vi "KepcoDCPwr Arbitrary Waveform.vi"(0 "VISA resource name":refnum<visa-resource-name>="GPIB0::3::INSTR", 1 "Open / Close":bool=TRUE, 5 "Model In":string, 11 "error in (no error)":errorcluster) -> (15 "error out":errorcluster)   [LabVIEW 2013]
panel:
  out "List not\nCorrected":bool
  out "list run":bool=TRUE
  out "Download time":u32
  out "Total time 2":dbl
  in  "CLR LIST":bool
  out "Total time":dbl=0.0015
  out "Measured Voltage Outptut":dbl(graph)=0.0646 caption="Current Measurements"
  in  "Load CSV":bool
  in  "List type":bool=TRUE
  out "Instrument Error":errorcluster
  in  "Start":bool caption="Downloading"
  in  "Exit":bool
  in  "Stop":bool
  in  "Protect":dbl caption="Voltage" min=0.0 max=20.0 step=1.0 format="%.2f"
  in  "Waveform List":string[][](table)=[["1", ".01"], ["2", ".01"], ["3", ".01"], ["4\n", ".01"], ["3", ".01"], ["2", ".01"], ["1", ".01"], ["0", ".01"]]
  in  "# of Cycles":i32=1
  in  "Disable @ End":bool
  out "Waveform Graph":T1(graph)={"Dwell (Sec)"=[0.0, 0.0005, 0.001, 0.0015], "Voltage Data"=[1.0, 2.0, 3.0]}
  out "number of points":i32=3 caption="Number of points"
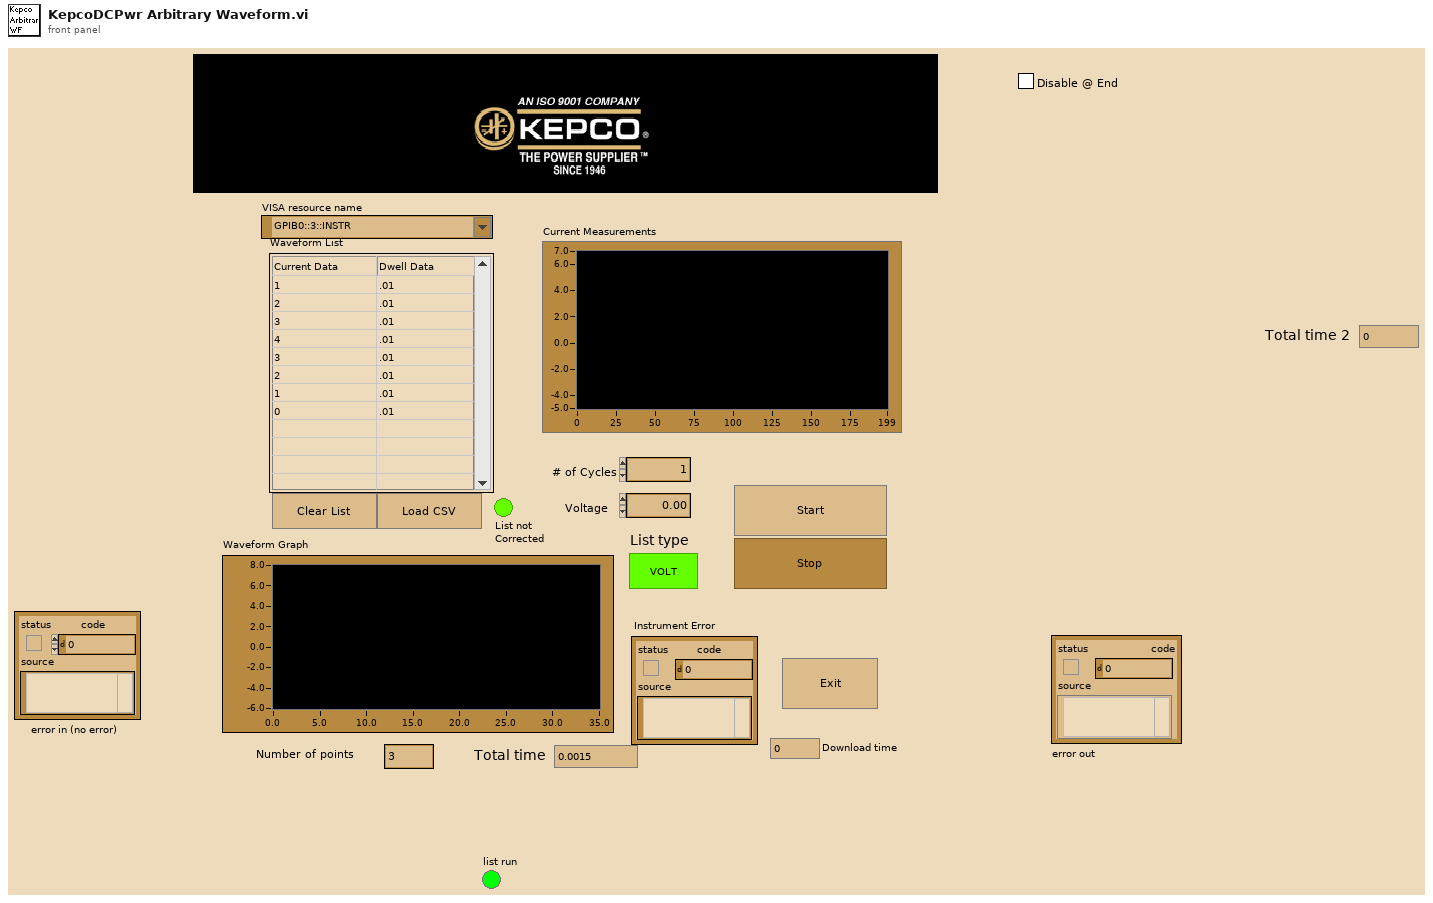
[diagram p1: front panel]
types:
  T1 = cluster{"Dwell (Sec)":dbl[], "Voltage Data":dbl[]}
  T2 = cluster{bool, "error code":i32, "error message":string}
  T3 = enum16{"Fixed", "List", "Transient", "External", "Gain", "Protect"}
  T4 = enum16{"open", "replace", "create", "open or create", "replace or create", "replace or create with confirmation"}
  T5 = cluster{"[0]":i32, "[1]":i32, "[2]":i32, "[3]":i32, "[4]":i32, "[5]":i32, "[6]":i32, "[7]":i32, "[8]":i32}
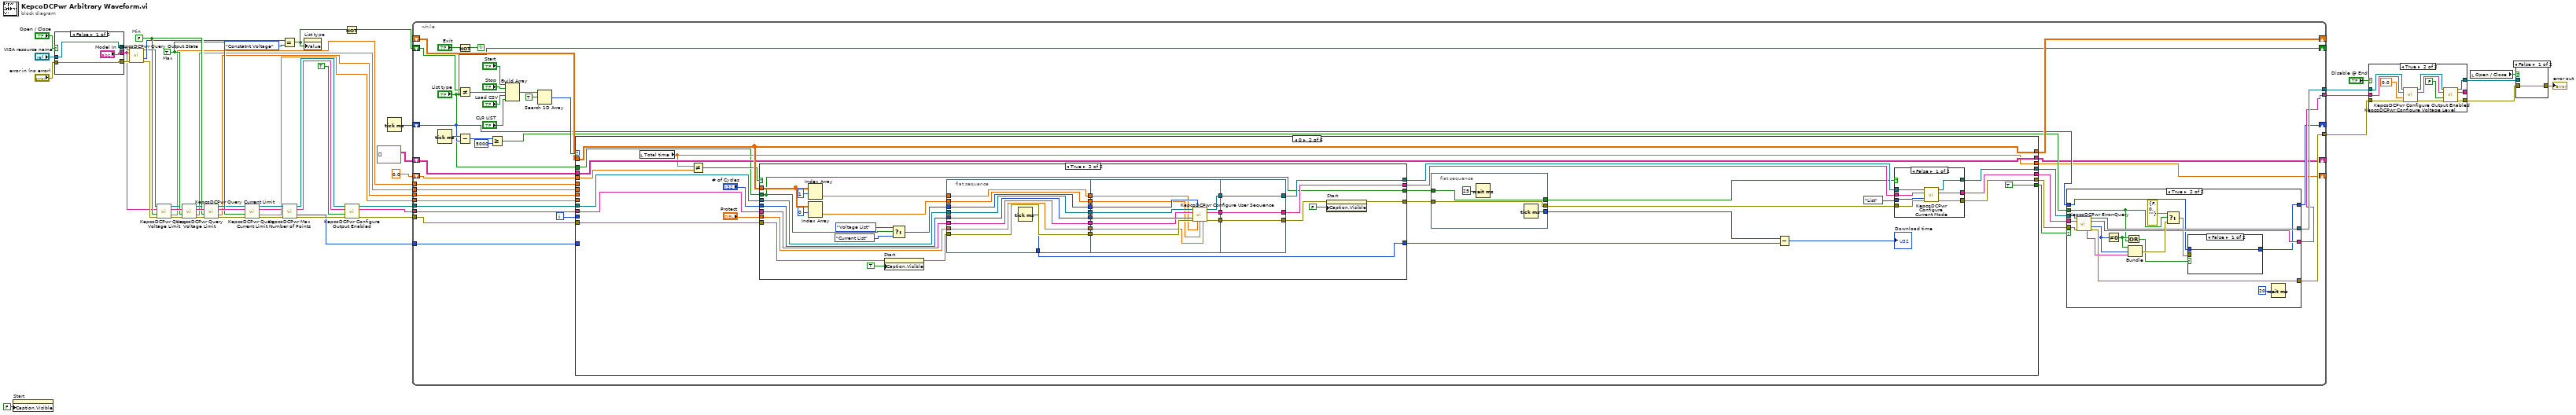
[diagram p0: block diagram]
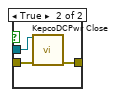
[diagram p2: hidden frame]
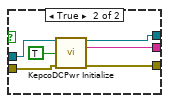
[diagram p3: hidden frame]
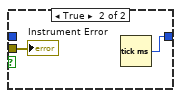
[diagram p5: hidden frame]
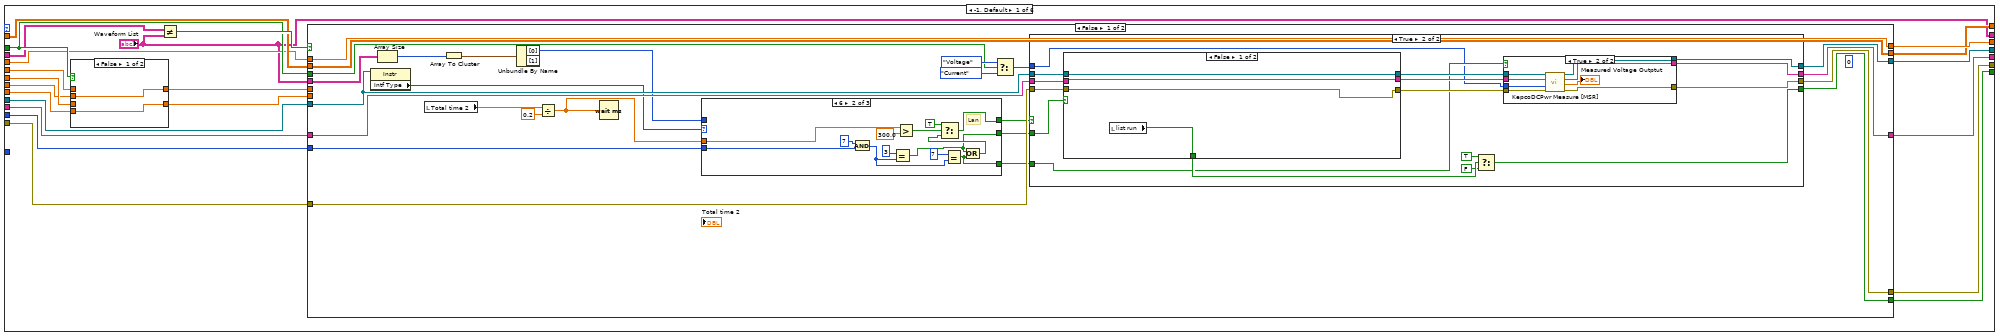
[diagram p6: hidden frame]
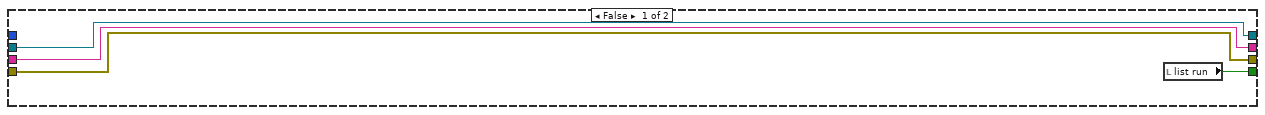
[diagram p8: hidden frame]
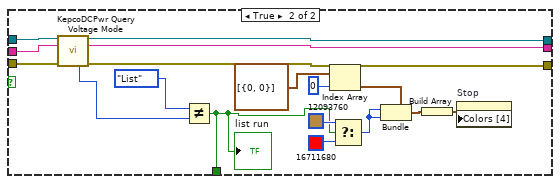
[diagram p9: hidden frame]
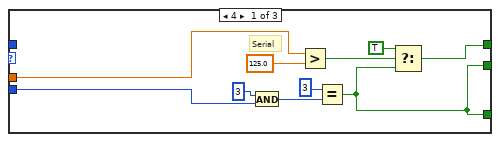
[diagram p11: hidden frame]
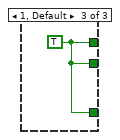
[diagram p12: hidden frame]
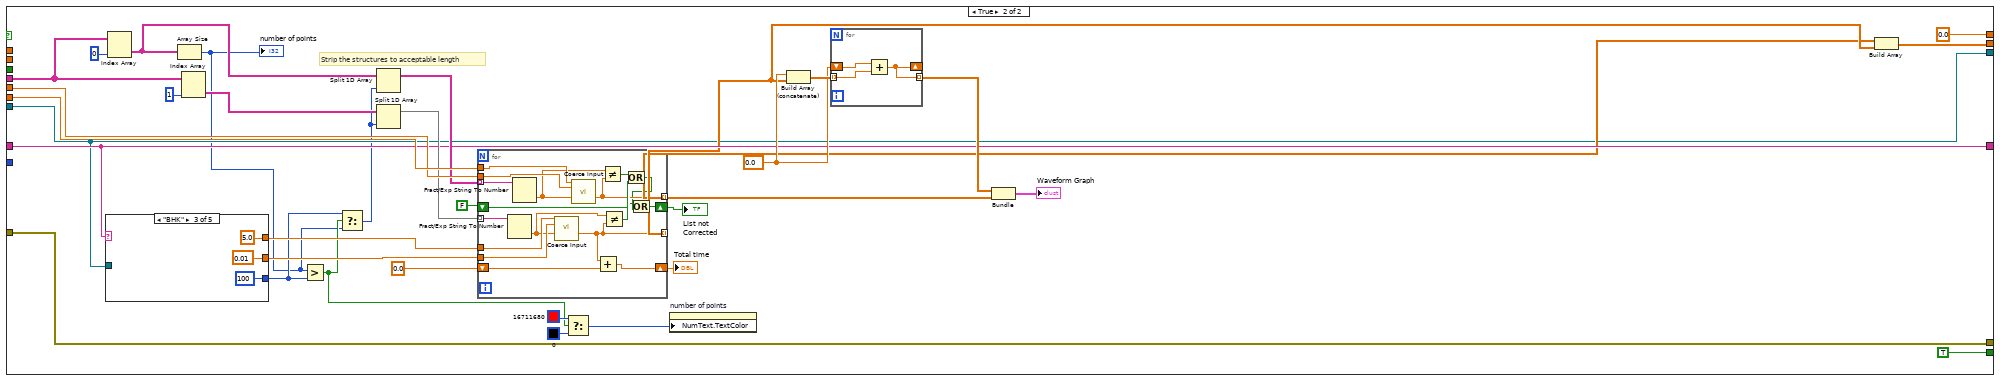
[diagram p13: hidden frame]
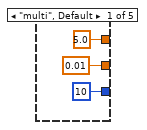
[diagram p14: hidden frame]
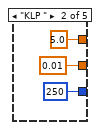
[diagram p15: hidden frame]
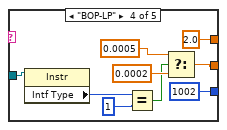
[diagram p16: hidden frame]
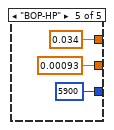
[diagram p17: hidden frame]
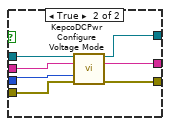
[diagram p18: hidden frame]
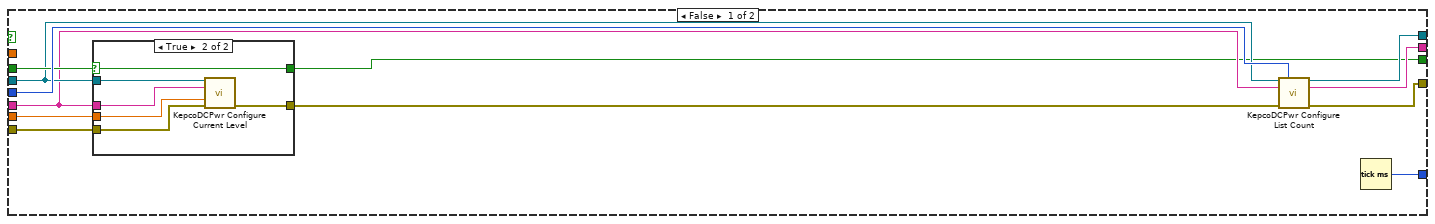
[diagram p19: hidden frame]
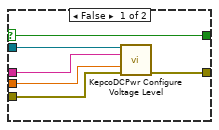
[diagram p20: hidden frame]
diagram:
  w26 = TRUE  # Max
  w27 = FALSE  # Min
  n1 = property on="Start" class="Bool"("Caption.Visible"=FALSE) -> ()  [unwired: 2 in, 2 out]
  n2 = case shown="False" "Open / Close" {
    tunnel: "error in (no error)" -> [w52 w58]
    tunnel: "VISA resource name" -> [w53 w57]
    tunnel: [w52 w56] -> w14
    tunnel: [w53 w55] -> w12
    tunnel: ["Model In" w54] -> w10
    frame False {
    }
    frame True {
      n3 = call "KepcoDCPwr Initialize.vi"("VISA Resource Name"=w57, "id query (True)"=TRUE, "error in (no error)"=w58) -> ("VISA Session Out"=w55:refnum<visa-resource-name>, "Model Out"=w54:string, "error out"=w56:errorcluster)  [unwired: 3 in, 7 out]
    }
  }
  n4 = call "KepcoDCPwr Query Output State.vi"("VISA Session"=w12, "Model In"=w10, "error in (no error)"=w14) -> ("VISA Session Out"=w11:refnum<visa-resource-name>, "Output state (Constant Voltage)"=w15:enum16{"Constatnt Voltage", "Constant Current"}, "error out"=w13:errorcluster)  [unwired: 5 in, 5 out]
  n5 = call "KepcoDCPwr Query Voltage Limit.vi"("VISA Session"=w11, "Model In"=w10, "Max Level (T),MIN LEVEL(F)"=w27, "error in (no error)"=w13) -> ("VISA Session Out"=w23:refnum<visa-resource-name>, "Model Out"=w32:string, "voltage level"=w17:dbl, "error out"=w33:errorcluster)  [unwired: 1 in, 7 out]
  n6 = call "KepcoDCPwr Query Voltage Limit.vi"("VISA Session"=w23, "Model In"=w32, "Max Level (T),MIN LEVEL(F)"=w26, "error in (no error)"=w33) -> ("VISA Session Out"=w24:refnum<visa-resource-name>, "Model Out"=w28:string, "voltage level"=w18:dbl, "error out"=w31:errorcluster)  [unwired: 1 in, 7 out]
  n7 = call "KepcoDCPwr Query Current Limit.vi"("VISA Session"=w24, "Model In"=w28, "Level"=w27, "error in (no error)"=w31) -> ("VISA Session Out"=w25:refnum<visa-resource-name>, "Model Out"=w29:string, "current limit"=w19:dbl, "error out"=w30:errorcluster)  [unwired: 1 in, 7 out]
  n8 = call "KepcoDCPwr Query Current Limit.vi"("VISA Session"=w25, "Model In"=w29, "Level"=w26, "error in (no error)"=w30) -> ("VISA Session Out"=w21:refnum<visa-resource-name>, "Model Out"=w7:string, "current limit"=w20:dbl, "error out"=w22:errorcluster)  [unwired: 1 in, 7 out]
  n9 = Equal?(x=w15, y=enum16{"Constatnt Voltage", "Constant Current"}."Constatnt Voltage" ("Output state (Constant Voltage)")) -> (x = y?=w9:bool)
  n10 = call "KepcoDCPwr Max Number of Points.vi"("VISA Session"=w21, "Model In"=w7, "error in (no error)"=w22) -> ("VISA Session Out"=w36:refnum<visa-resource-name>, "Model Out"=w34:string, "Max # of Pts"=w1:i32, "error out"=w35:errorcluster)  [unwired: 1 in, 8 out]
  n11 = property on="List type" class="Bool (strict)"("Value"=w9) -> ()  [unwired: 2 in, 2 out]
  n12 = Not(x=w9) -> (.not. x?=w8:bool)
  n13 = call "KepcoDCPwr Configure Output Enabled.vi"("VISA Session"=w36, "Model In"=w34, "Input enabled (True)"=TRUE, "error in (no error)"=w35) -> ("VISA Session Out"=w46:refnum<visa-resource-name>, "Model Out"=w45:string, "error out"=w44:errorcluster)  [unwired: 9 out]
  n14 = Tick Count (ms)() -> (millisecond timer value=w38:u32)
  n15 = while {
    shift-left: w38 -> [w78]
    shift-right: [w76] -> _
    shift-left: _ -> [w92]
    shift-right: [w91] -> _
    tunnel: w44 -> [w98]
    tunnel: [w82] -> w41
    tunnel: w45 -> [w97]
    tunnel: [w81] -> w42
    tunnel: w46 -> [w96]
    tunnel: [w83] -> w43
    shift-right: ["List type"] -> _
    shift-left: w8 -> [w75]
    tunnel: w19 -> [w71]
    tunnel: w20 -> [w70]
    tunnel: w18 -> [w72]
    tunnel: w17 -> [w73]
    shift-right: [w69] -> _
    shift-left: string[][] [] ("Data Table") -> [w68]
    shift-right: [w65] -> _
    shift-left: 0.0 ("Total time") -> [w64]
    tunnel: w1 -> [w60]
    i -> [w62]
    stop <- w99 continue-if-true
    n16 = Tick Count (ms)() -> (millisecond timer value=w87:u32)
    n17 = Not(x="Exit") -> (.not. x?=w99:bool)
    n18 = Not Equal?(x=w75, y="List type") -> (x != y?=w74:bool)
    n19 = Subtract(x=w87, y=w78) -> (x-y=w86:u32)
    n20 = Greater Or Equal?(x=w86, y=u32 5000) -> (x >= y?=w77:bool)
    n21 = Build Array("Start", "Stop", w74, "Load CSV", "CLR LIST") -> (w95:bool[])
    n22 = Search 1D Array(1D array=w95, element=TRUE) -> (index of element=w94:i32)  [unwired: 1 in]
    n23 = case shown="0" w94 {
      tunnel: w96 -> [w142 w342 w468 w501 w519 w542]
      tunnel: w97 -> [w141 w343 w467 w499 w520 w540]
      tunnel: w98 -> [w140 w344 w451 w498 w521 w538]
      tunnel: [w138 w349 w468 w500 w519 w541] -> w84
      tunnel: w92 -> [w144 w345 w469 w495 w524 w546]
      tunnel: [w136 w345 w469 w495 w524 w546] -> w91
      tunnel: [w139 w333 w450 w496 w521 w537] -> w80
      tunnel: [w137 w350 w467 w497 w520 w539] -> w79
      tunnel: w73 -> [w134 _ _ _ _ w536]
      tunnel: w72 -> [w133 _ _ _ _ w535]
      tunnel: w71 -> [w132 _ _ _ _ w533]
      tunnel: w70 -> [w131 _ _ _ _ w532]
      tunnel: ["Waveform List" w341 w453 w494 w523 string[][] [] ("Data Table")] -> w69
      tunnel: w68 -> [w126 w341 w453 w494 w523 _]
      tunnel: "List type" -> [w135 w336 _ w492 _ w529]
      tunnel: [w143 w340 w452 w493 w522 w531] -> w65
      tunnel: w64 -> [w128 w339 w452 w493 w522 w531]
      tunnel: w62 -> [w125 _ _ _ _ _]
      tunnel: [w124 TRUE _ TRUE TRUE TRUE] -> w61
      tunnel: w60 -> [_ _ _ _ _ _]
      frame -1, Default {
        n24 = case shown="False" w135 {
          tunnel: w134 -> [_ w149]
          tunnel: w133 -> [_ w148]
          tunnel: w132 -> [w147 _]
          tunnel: w131 -> [w146 _]
          tunnel: [w147 w149] -> w129
          tunnel: [w146 w148] -> w130
          frame False {
          }
          frame True {
          }
        }
        n25 = Not Equal?(x=w126, y="Waveform List") -> (x != y?=w145:bool)
        n26 = case shown="False" w145 {
          tunnel: [w174 w259] -> w136
          tunnel: w130 -> [_ w284]
          tunnel: w129 -> [_ w283]
          tunnel: "Waveform List" -> [w160 w267]
          tunnel: w144 -> [w174 _]
          tunnel: [w163 0.0 ("Total time")] -> w143
          tunnel: w135 -> [w171 _]
          tunnel: w142 -> [w162 w255]
          tunnel: w141 -> [w170 w264]
          tunnel: w140 -> [w169 w265]
          tunnel: [w167 w265] -> w139
          tunnel: [w166 w255] -> w138
          tunnel: [w165 w264] -> w137
          tunnel: w128 -> [w163 _]
          tunnel: w125 -> [w155 _]
          tunnel: [w152 TRUE] -> w124
          frame False {
            (unwired) 0 ("y")
            n27 = property class="Instr"(reference=w162) -> ("Intf Type"=w161:u16)  [unwired: 1 in, 2 out]
            n28 = Array Size(array=w160) -> (size(s)=w159:i32[])
            n29 = local read "Total time 2"() -> (w164:dbl)
            n30 = Array To Cluster(array=w159) -> (cluster=w158:T5)
            n31 = Unbundle By Name(w158) -> ("[0]"=w157:i32)  [unwired: 1 out]
            n32 = Divide(x=w164, y=0.2) -> (x/y=w153:dbl)
            n33 = Wait (ms)(milliseconds to wait=w153) -> ()  [unwired: 1 out]
            n34 = case shown="6" w161 {
              tunnel: w157 -> [_ _ _]
              tunnel: [w229 w243 w250] -> w156
              tunnel: w155 -> [w236 w249 _]
              tunnel: w153 -> [w232 w246 _]
              tunnel: [w227 w238 w250] -> w151
              tunnel: [w227 w237 w250] -> w150
              frame 4 {
                # "Serial"
                n35 = And(x=3, y=w236) -> (x .and. y?=w234:i32)
                n36 = Greater?(x=w232, y=125.0) -> (0:w230:bool)
                n37 = Equal?(x=3, y=w234) -> (x = y?=w227:bool)
                n38 = Select(t=TRUE, s=w230, f=w227) -> (s? t:f=w229:bool)
              }
              frame 6 {
                # "Lan"
                n39 = And(x=7, y=w249) -> (x .and. y?=w241:i32)
                n40 = Equal?(x=3, y=w241) -> (x = y?=w238:bool)
                n41 = Greater?(x=w246, y=300.0) -> (0:w244:bool)
                n42 = Equal?(x=7, y=w241) -> (x = y?=w237:bool)
                n43 = Or(x=w238, y=w237) -> (x .or. y?=w239:bool)
                n44 = Select(t=TRUE, s=w244, f=w239) -> (s? t:f=w243:bool)
              }
              frame 1, Default {
                w250 = TRUE
              }
            }
            n45 = Select(t=enum16{"Voltage", "Current"}."Voltage" ("measurement type (voltage)"), s=w171, f=enum16{"Voltage", "Current"}."Current") -> (s? t:f=w168:enum16{"Voltage", "Current"})
            n46 = case shown="True" w156 {
              tunnel: w170 -> [w177 w191]
              tunnel: w169 -> [w176 w190]
              tunnel: w168 -> [_ w179]
              tunnel: [w176 w189] -> w167
              tunnel: [w178 w188] -> w166
              tunnel: [w177 w187] -> w165
              tunnel: w162 -> [w178 w186]
              tunnel: [w175 w183] -> w152
              tunnel: w151 -> [_ w181]
              tunnel: w150 -> [_ w180]
              frame False {
                n47 = local read "list run"() -> (w175:bool)
              }
              frame True {
                n48 = case shown="False" w181 {
                  tunnel: [w196 w207] -> w194
                  tunnel: [w195 w206] -> w193
                  tunnel: [w197 w205] -> w192
                  tunnel: w191 -> [w196 w204]
                  tunnel: w190 -> [w197 w203]
                  tunnel: w186 -> [w195 w202]
                  tunnel: [w198 w199] -> w185
                  frame False {
                    n49 = local read "list run"() -> (w198:bool)
                  }
                  frame True {
                    n50 = call "KepcoDCPwr Query Voltage Mode.vi"("VISA Session"=w202, "Model In"=w204, "error in (no error)"=w203) -> ("VISA Session Out"=w206:refnum<visa-resource-name>, "Model Out"=w207:string, "Mode (Fixed)"=w201:T3, "error out"=w205:errorcluster)  [unwired: 1 in, 8 out]
                    n51 = Not Equal?(x=T3."List", y=w201) -> (x != y?=w199:bool)
                    "list run" <- w199
                    n52 = Index Array(array=cluster{u32, u32}[] [{0, 0}] ("Colors [4]"), index=0) -> (element=w213:cluster{u32, u32})
                    n53 = Select(t=u32 12093760, s=w199, f=u32 16711680) -> (s? t:f=w210:u32)
                    n54 = Bundle(cluster=w213, w210, w210) -> (w212:cluster{u32, u32})
                    n55 = Build Array(w212) -> (w215:cluster{u32, u32}[])
                    n56 = property on="Stop" class="Bool"("Colors [4]"=w215) -> ()  [unwired: 2 in, 2 out]
                  }
                }
                n57 = Select(t=TRUE, s=w185, f=FALSE ("x != y?")) -> (s? t:f=w183:bool)
                n58 = case shown="True" w180 {
                  tunnel: w194 -> [w216 w226]
                  tunnel: w193 -> [w217 w225]
                  tunnel: w192 -> [w218 w224]
                  tunnel: w179 -> [_ w223]
                  tunnel: [w218 w221] -> w189
                  tunnel: [w217 w220] -> w188
                  tunnel: [w216 w219] -> w187
                  frame False {
                  }
                  frame True {
                    n59 = call "KepcoDCPwr Measure [MSR].vi"("VISA Session"=w225, "Model In"=w226, "measurement type (voltage)"=w223, "error in (no error)"=w224) -> ("VISA Session Out"=w220:refnum<visa-resource-name>, "Model Out"=w219:string, "measurement"=→"Measured Voltage Outptut":dbl, "error out"=w221:errorcluster)  [unwired: 4 in, 4 out]
                  }
                }
              }
            }
          }
          frame True {
            w279 = 0.0
            # "Strip the structures to acceptable length"
            n60 = case shown="\"BHK\"" w264 {
              tunnel: [5.0 5.0 5.0 2.0 0.034] -> w263
              tunnel: [0.01 0.01 0.01 w297 0.00093] -> w262
              tunnel: [10 250 100 1002 5900] -> w253
              tunnel: w255 -> [_ _ _ w300 _]
              frame "multi", Default {
              }
              frame "KLP " {
              }
              frame "BHK" {
              }
              frame "BOP-LP" {
                n61 = property class="Instr"(reference=w300) -> ("Intf Type"=w295:u16)  [unwired: 1 in, 2 out]
                n62 = Equal?(x=w295, y=u16 1 ("x")) -> (x = y?=w296:bool)
                n63 = Select(t=0.0005, s=w296, f=0.0002) -> (s? t:f=w297:dbl)
              }
              frame "BOP-HP" {
              }
            }
            n64 = Index Array(array=w267, index (col)=0) -> (element=w266:string[])  [unwired: 1 in]
            n65 = Array Size(array=w266) -> (size(s)=w252:i32)
            "number of points" <- w252
            n66 = Index Array(array=w267, index (col)=1) -> (element=w275:string[])  [unwired: 1 in]
            n67 = Greater?(x=w252, y=w253) -> (0:w254:bool)
            n68 = Select(t=w253, s=w254, f=w252) -> (s? t:f=w251:i32)
            n69 = Split 1D Array(array=w266, index=w251) -> (first subarray=w276:string[])  [unwired: 1 out]
            n70 = Split 1D Array(array=w275, index=w251) -> (first subarray=w274:string[])  [unwired: 1 out]
            n71 = for {
              tunnel: w276 -> [w322] mode=indexing
              tunnel: [w312] -> w260 mode=indexing
              tunnel: w274 -> [w321] mode=indexing
              tunnel: [w311] -> w261 mode=indexing
              tunnel: w284 -> [w313]
              tunnel: w283 -> [w320]
              shift-right: [w319] -> w272
              shift-left: 0.0 -> [w318]
              tunnel: w263 -> [w317]
              tunnel: w262 -> [w316]
              shift-right: [w306] -> w256
              shift-left: FALSE -> [w307]
              n72 = Fract/Exp String To Number(string=w321) -> (number=w309:dbl)  [unwired: 4 out]
              n73 = Fract/Exp String To Number(string=w322) -> (number=w310:dbl)  [unwired: 4 out]
              n74 = call "Coerce Input.vi"("Max"=w317, "Min"=w316, "Input"=w309) -> ("Output"=w311:dbl)  [unwired: 12 out]
              n75 = call "Coerce Input.vi"("Max"=w313, "Min"=w320, "Input"=w310) -> ("Output"=w312:dbl)  [unwired: 12 out]
              n76 = Add(x=w311, y=w318) -> (x+y=w319:dbl)
              n77 = Not Equal?(x=w310, y=w312) -> (x != y?=w315:bool)
              n78 = Not Equal?(x=w309, y=w311) -> (x != y?=w314:bool)
              n79 = Or(x=w315, y=w314) -> (x .or. y?=w308:bool)
              n80 = Or(x=w307, y=w308) -> (x .or. y?=w306:bool)
            }
            "Total time" <- w272
            "List not\nCorrected" <- w256
            n81 = Select(t=u32 16711680, s=w254, f=u32 0) -> (s? t:f=w270:u32)
            n82 = property on="number of points" class="DigNum (strict)"("NumText.TextColor"=w270) -> ()  [unwired: 2 in, 2 out]
            n83 = Build Array (concatenate)(w279, w261) -> (w280:dbl[])
            n84 = for {
              tunnel: w280 -> [w325] mode=indexing
              shift-right: [w323] -> _
              shift-left: w279 -> [w324]
              tunnel: [w323] -> w281 mode=indexing
              n85 = Add(x=w324, y=w325) -> (x+y=w323:dbl)
            }
            n86 = Bundle(w281, w260) -> (→"Waveform Graph":cluster{dbl[], dbl[]})  [unwired: 1 out]
            n87 = Build Array(w260, w261) -> (w259:dbl[][])
          }
        }
      }
      frame 0 {
        n88 = local read "Total time"() -> (w340:dbl)
        n89 = Not Equal?(x=w340, y=w339) -> (x != y?=w338:bool)
        n90 = case shown="True" w338 {
          tunnel: [w376 w421] -> w348
          tunnel: [w375 w420] -> w347
          tunnel: [w374 w413] -> w335
          tunnel: "# of Cycles" -> [w373 w419]
          tunnel: w345 -> [_ w405]
          tunnel: w344 -> [w368 w416]
          tunnel: w343 -> [w369 w418]
          tunnel: w342 -> [w370 w417]
          tunnel: "Protect" -> [w372 w410]
          tunnel: w336 -> [w371 w389]
          tunnel: [w366 w390] -> w330
          tunnel: [w365 w389] -> w328
          frame False {
            n91 = case shown="True" w371 {
              selector: w371 -> [w377 w383]
              tunnel: w372 -> [w382 w388]
              tunnel: w370 -> [w381 w387]
              tunnel: w369 -> [w380 w386]
              tunnel: w368 -> [w379 w384]
              tunnel: [w378 w385] -> w367
              tunnel: [w377 w383] -> w365
              frame False {
                n92 = call "KepcoDCPwr Configure Voltage Level.vi"("VISA Session"=w381, "Model In"=w380, "level (0.0 volts)"=w382, "error in (no error)"=w379) -> ("error out"=w378:errorcluster)  [unwired: 8 in, 3 out]
              }
              frame True {
                n93 = call "KepcoDCPwr Configure Current Level.vi"("VISA Session"=w387, "Model In"=w386, "level (0.0 volts)"=w388, "error in (no error)"=w384) -> ("error out"=w385:errorcluster)  [unwired: 8 in, 3 out]
              }
            }
            n94 = call "KepcoDCPwr Configure List Count.vi"("VISA Session"=w370, "# of Cycles"=w373, "Model In"=w369, "error in (no error)"=w367) -> ("VISA Session Out"=w376:refnum<visa-resource-name>, "Model Out"=w375:string, "error out"=w374:errorcluster)  [unwired: 8 in, 1 out]
            n95 = Tick Count (ms)() -> (millisecond timer value=w366:u32)
          }
          frame True {
            n96 = Index Array(array=w405, index (row)=1 ("index")) -> (element=w406:dbl[])  [unwired: 1 in]
            n97 = Index Array(array=w405, index (row)=0 ("index")) -> (element=w404:dbl[])  [unwired: 1 in]
            n98 = property on="Start" class="Bool"(error in=w416, "Caption.Visible"=TRUE) -> (error out=w415:errorcluster)  [unwired: 1 in, 1 out]
            n99 = Select(t=enum16{"Current List", "Voltage List"}."Voltage List" ("List Mode (volt/current)"), s=w389, f=enum16{"Current List", "Voltage List"}."Current List") -> (s? t:f=w408:enum16{"Current List", "Voltage List"})
            n100 = flat-sequence {
              tunnel: w404 -> [w423]
              tunnel: w406 -> [w424]
              tunnel: w408 -> [w425]
              tunnel: w410 -> [w426]
              tunnel: w415 -> [w427]
              tunnel: w417 -> [w428]
              tunnel: w418 -> [w429]
              tunnel: w419 -> [w430]
              tunnel: [w430] -> w398
              tunnel: [w429] -> w397
              tunnel: [w428] -> w396
              tunnel: [w427] -> w395
              tunnel: [w426] -> w394
              tunnel: [w425] -> w393
              tunnel: [w424] -> w392
              tunnel: [w423] -> w391
              tunnel: [w422] -> w390
              tunnel: [w441] -> w401
              tunnel: [w440] -> w400
              tunnel: [w435] -> w399
              tunnel: w398 -> [w439]
              tunnel: w397 -> [w438]
              tunnel: w396 -> [w437]
              tunnel: w395 -> [w436]
              tunnel: w394 -> [w434]
              tunnel: w393 -> [w433]
              tunnel: w392 -> [w432]
              tunnel: w391 -> [w431]
              tunnel: [w442] -> w412
              tunnel: [w443] -> w420
              tunnel: [w444] -> w421
              tunnel: w401 -> [w444]
              tunnel: w400 -> [w443]
              tunnel: w399 -> [w442]
              frame #0 {
                n101 = Tick Count (ms)() -> (millisecond timer value=w422:u32)
              }
              frame #1 {
                n102 = call "KepcoDCPwr Configure User Sequence.vi"("VISA Session"=w437, "List Mode (volt/current)"=w433, "Model In"=w438, "# of Cycles"=w439, "error in (no error)"=w436, "Dwell (sec)"=w432, "List Data"=w431, "Limit Value"=w434) -> ("VISA Session Out"=w441:refnum<visa-resource-name>, "Model Out"=w440:string, "error out"=w435:errorcluster)  [unwired: 1 in, 4 out]
              }
              frame #2 {
              }
            }
            n103 = property on="Start" class="Bool"(error in=w412, "Caption.Visible"=FALSE) -> (error out=w413:errorcluster)  [unwired: 1 in, 1 out]
          }
        }
        n104 = flat-sequence {
          tunnel: [w447] -> w334
          tunnel: w335 -> [w447]
          tunnel: [w446] -> w332
          tunnel: [w445] -> w329
          tunnel: w328 -> [w445]
          frame #0 {
            n105 = Wait (ms)(milliseconds to wait=u32 25) -> ()  [unwired: 1 out]
            n106 = Tick Count (ms)() -> (millisecond timer value=w446:u32)
          }
        }
        n107 = Subtract(x=w332, y=w330) -> (x-y=→"Download time":u32)
        n108 = case shown="False" w329 {
          tunnel: [w352 w364] -> w350
          tunnel: [w351 w363] -> w349
          tunnel: w348 -> [w357 w362]
          tunnel: w347 -> [w356 w361]
          tunnel: w334 -> [w355 w360]
          tunnel: [w353 w359] -> w333
          tunnel: T3."List" ("Mode (Fixed)") -> [w354 w358]
          frame False {
            n109 = call "KepcoDCPwr Configure Current Mode.vi"("VISA Session"=w357, "Model In"=w356, "Mode (Fixed)"=w354, "error in (no error)"=w355) -> ("VISA Session Out"=w351:refnum<visa-resource-name>, "Model Out"=w352:string, "error out"=w353:errorcluster)  [unwired: 8 in, 1 out]
          }
          frame True {
            n110 = call "KepcoDCPwr Configure Voltage Mode.vi"("VISA Session"=w362, "Model In"=w361, "Mode (Fixed)"=w358, "error in (no error)"=w360) -> ("VISA Session Out"=w363:refnum<visa-resource-name>, "Model Out"=w364:string, "error out"=w359:errorcluster)  [unwired: 2 in, 7 out]
          }
        }
      }
      frame 3 {
        n111 = Open/Create/Replace File(error in=w451, prompt="Select txt or csv file", operation (0:open)=T4."open", access (0:read/write)=enum16{"read/write", "read-only", "write-only"}."read-only") -> (refnum out=w461:refnum<file>, error out=w462:errorcluster)  [unwired: 2 in, 1 out]
        n112 = Get File Size(file=w461, error in=w462) -> (size (in bytes)=w456:i64, 0:w457:errorcluster)  [unwired: 1 out]
        n113 = while {
          tunnel: w461 -> [w477]
          tunnel: [w476] -> w460
          tunnel: [w471] -> w458
          tunnel: w457 -> [w470]
          stop <- w472 stop-if-true
          n114 = Read from Text File(file (use dialog)=w477, error in=w470) -> (refnum out=w476:refnum<file>, text=w475:string, error out=w471:errorcluster)  [unwired: 2 in, 1 out]
          n115 = Match Pattern(string=w475, regular expression="\"") -> (offset past match=w473:i32)  [unwired: 1 in, 3 out]
          n116 = Less Than 0?(x=w473) -> (x < 0?=w472:bool)
        }
        n117 = Subtract(x=w456, y=i64 5) -> (x-y=w454:i64)
        n118 = while {
          tunnel: w460 -> [w490]
          tunnel: [w485] -> w463
          tunnel: [w483] -> w459
          tunnel: w458 -> [w482]
          tunnel: w454 -> [w481]
          tunnel: [w478] -> w449 mode=indexing
          stop <- w487 stop-if-true
          n119 = Read from Text File(file (use dialog)=w490, error in=w482) -> (refnum out=w485:refnum<file>, text=w489:string, error out=w484:errorcluster)  [unwired: 2 in, 1 out]
          n120 = Get File Position(4:w484, 7:w485) -> (0:w483:errorcluster, 2:w486:i64)  [unwired: 1 out]
          n121 = Match Pattern(string=w489, regular expression="\t") -> (before substring=w480:string, after substring=w479:string)  [unwired: 1 in, 2 out]
          n122 = Greater?(x=w486, y=w481) -> (0:w487:bool)
          n123 = Build Array(w480, w479) -> (w478:string[])
        }
        n124 = local write "Waveform List"(w449) -> ()
        n125 = Close File(refnum=w463, error in=w459) -> (error out=w450:errorcluster)  [unwired: 1 out]
      }
      frame 1 {
        n126 = case shown="False" w492 {
          tunnel: T3."Fixed" ("Mode (Fixed)") -> [w509 w516]
          tunnel: w501 -> [w508 w515]
          tunnel: [w507 w514] -> w500
          tunnel: w499 -> [w506 w513]
          tunnel: w498 -> [w505 w512]
          tunnel: [w504 w511] -> w497
          tunnel: [w503 w510] -> w496
          frame False {
            n127 = call "KepcoDCPwr Configure Current Mode.vi"("VISA Session"=w508, "Model In"=w506, "Mode (Fixed)"=w509, "error in (no error)"=w505) -> ("VISA Session Out"=w507:refnum<visa-resource-name>, "Model Out"=w504:string, "error out"=w503:errorcluster)  [unwired: 8 in, 1 out]
          }
          frame True {
            n128 = call "KepcoDCPwr Configure Voltage Mode.vi"("VISA Session"=w515, "Model In"=w513, "Mode (Fixed)"=w516, "error in (no error)"=w512) -> ("VISA Session Out"=w514:refnum<visa-resource-name>, "Model Out"=w511:string, "error out"=w510:errorcluster)  [unwired: 2 in, 7 out]
          }
        }
      }
      frame 4 {
        # "Clear the waveform list"
        n129 = local write "Waveform List"(string[][] [["1", ".1"], ["2", ".1"]] ("Waveform List")) -> ()
      }
      frame 2 {
        # "List mode change"
        n130 = case shown="True" w529 {
          tunnel: w536 -> [_ _]
          tunnel: w535 -> [w550 _]
          tunnel: [w550 w554] -> w534
          tunnel: w533 -> [_ _]
          tunnel: w532 -> [_ w554]
          tunnel: ["Voltage" ("new element/subarray") "Current" ("f")] -> w528
          tunnel: ["Current Measurements" ("f") "Voltage Measurements" ("f")] -> w527
          tunnel: ["Current Data" ("f") "Voltage Data" ("new element/subarray")] -> w526
          frame False {
          }
          frame True {
          }
        }
        n131 = property on="Waveform List" class="Tbl (strict)"() -> ("Column Headers[]"=w545:string[])  [unwired: 2 in, 2 out]
        n132 = property on="Measured Voltage Outptut" class="WFChart (strict)"("Caption.Text"=w527) -> ()  [unwired: 2 in, 2 out]
        n133 = property on="Protect" class="DigNum (strict)"("Caption.Text"=w528, "Maximum"=w534) -> ()  [unwired: 2 in, 2 out]
        n134 = Replace Array Subset(array=w545, new element=w526, index=0) -> (w543:string[])
        n135 = property on="Waveform List" class="Tbl (strict)"("Column Headers[]"=w543) -> ()  [unwired: 2 in, 2 out]
        n136 = call "KepcoDCPwr Configure Output State.vi"("VISA Session"=w542, "Model In"=w540, "Power Supply Mode"=w529, "error in (no error)"=w538) -> ("VISA Session Out"=w541:refnum<visa-resource-name>, "channel name out (\"\")"=w539:string, "error out"=w537:errorcluster)  [unwired: 8 in, 1 out]
      }
    }
    n137 = case shown="True" w61 {
      tunnel: w84 -> [w103 w113]
      tunnel: [w103 w112] -> w83
      tunnel: [w100 w111] -> w82
      tunnel: [w101 w110] -> w81
      tunnel: w80 -> [w100 w109]
      tunnel: w79 -> [w101 w108]
      tunnel: w78 -> [w102 w107]
      tunnel: w77 -> [_ w106]
      tunnel: [w102 w105] -> w76
      frame False {
      }
      frame True {
        n138 = call "KepcoDCPwr Error-Query.vi"("VISA Session"=w113, "Model In"=w108, "error in (no error)"=w109) -> ("VISA Session Out"=w112:refnum<visa-resource-name>, "Model Out"=w110:string, "error code"=w116:i32, "error message"=w115:string, "error out"=w111:errorcluster)  [unwired: 1 in, 7 out]
        n139 = Not Equal To 0?(x=w116) -> (x != 0?=w117:bool)
        n140 = Or(x=w117, y=w106) -> (x .or. y?=w114:bool)
        n141 = Bundle(w117, "error code"=w116, "error message"=w115) -> (w118:T2)  [unwired: 1 out]
        n142 = Select(t=T2 {FALSE, "error code"=0, "error message"=""}, s=w106, f=w118) -> (s? t:f=w119:T2)
        n143 = case shown="False" w114 {
          tunnel: [w121 w123] -> w105
          tunnel: w107 -> [w121 _]
          tunnel: w119 -> [_ w122]
          frame False {
          }
          frame True {
            n144 = Tick Count (ms)() -> (millisecond timer value=w123:u32)
            "Instrument Error" <- w122
          }
        }
        n145 = Wait (ms)(milliseconds to wait=u32 20) -> ()  [unwired: 1 out]
      }
    }
  }
  n146 = case shown="True" "Disable @ End" {
    tunnel: w43 -> [w557 w568]
    tunnel: w42 -> [w556 w567]
    tunnel: w41 -> [w555 w566]
    tunnel: [w555 w561] -> w49
    tunnel: [w557 w560] -> w50
    tunnel: [w556 w559] -> _
    frame False {
    }
    frame True {
      n147 = call "KepcoDCPwr Configure Voltage Level.vi"("VISA Session"=w568, "Model In"=w567, "level (0.0 volts)"=0.0, "error in (no error)"=w566) -> ("VISA Session Out"=w564:refnum<visa-resource-name>, "Model Out"=w563:string, "error out"=w562:errorcluster)  [unwired: 1 in, 8 out]
      n148 = call "KepcoDCPwr Configure Output Enabled.vi"("VISA Session"=w564, "Model In"=w563, "Input enabled (True)"=FALSE ("output enabled (True)"), "error in (no error)"=w562) -> ("VISA Session Out"=w560:refnum<visa-resource-name>, "Model Out"=w559:string, "error out"=w561:errorcluster)  [unwired: 9 out]
    }
  }
  n149 = local read "Open / Close"() -> (w2:bool)
  n150 = case shown="False" w2 {
    tunnel: w50 -> [_ w572]
    tunnel: w49 -> [w569 w571]
    tunnel: [w569 w570] -> w47
    frame False {
    }
    frame True {
      n151 = call "KepcoDCPwr Close.vi"("VISA Session"=w572, "error in (no error)"=w571) -> ("error out"=w570:errorcluster)  [unwired: 13 out]
    }
  }
  "error out" <- w47
